vi "Test_HelloWorld_InvalidUtf8Encoding.vi"() -> (0 "Array of Error Description":T1)   [LabVIEW 2019]
uses:
  gRPC_ATS/TestUtility/utility.llb/array of error description.ctl
  gRPC_ATS/TestUtility/utility.llb/error description.ctl
  gRPC_ATS/TestUtility/utility.llb/error type.ctl
  examples/helloworld/helloworld_client/RPC Messages/helloworld_HelloRequest.ctl
  690210b7-9fc1-4805-899f-f09b8e1640af.vi
  86c0777a-bec3-4a03-9553-2f9525a5fa02.vi
  <vilib>/gRPC/LabVIEW gRPC Library/Server API/Translate Protobuf Error.vi
  <vilib>/AdvancedString/1D String Array to Delimited String.vi
  <vilib>/gRPC/LabVIEW gRPC Library/Server API/Server/Get Server DLL Path.vi
  examples/helloworld/helloworld_client/helloworld_client.lvlib
panel:
  out "Pass":bool
  in  "error in (no error)":errorcluster
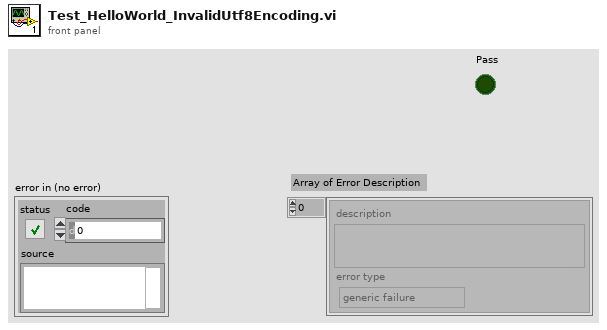
[diagram p1: front panel]
types:
  T1 = typedef "array of error description.ctl" = T2[]
  T2 = typedef "error description.ctl" = cluster{"description":string, "error type":T3}
  T3 = typedef "error type.ctl" = enum32{"generic failure", "boundary case", "precision", "expected error"}
  T4 = typedef "helloworld_client.lvlib/helloworld_HelloRequest.ctl" = cluster{"name":string}
  T5 = typedef "grpc-lvsupport-release.lvlib/grpcId.ctl" = u64
  T6 = typedef "grpc-lvsupport-release.lvlib/Any.ctl" = cluster{"Type Url":string, "Bytes":u8[]}
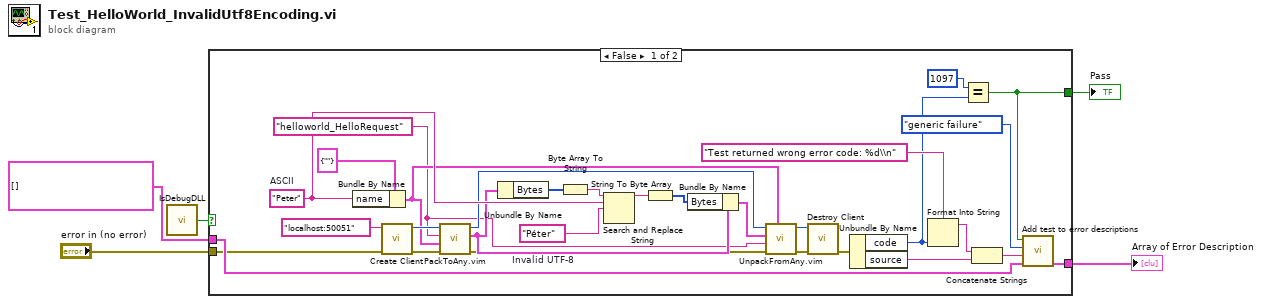
[diagram p0: block diagram]
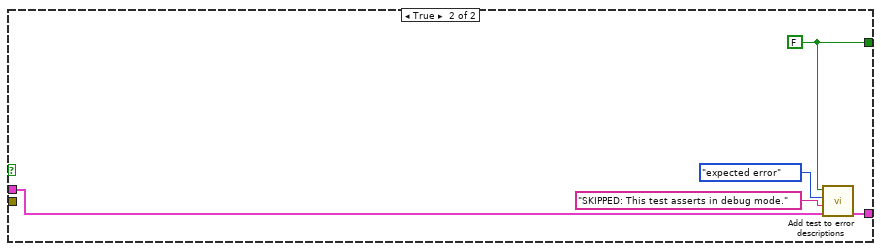
[diagram p2: hidden frame]
diagram:
  n1 = call "IsDebugDLL.vi"() -> ("is debug DLL?"=w1:bool)
  n2 = case shown="False" w1 {
    tunnel: T1 [] ("error descriptions in") -> [w35 w40]
    tunnel: [w34 w39] -> w4
    tunnel: "error in (no error)" -> [w13 _]
    tunnel: [w6 w36] -> w2
    frame False {
      w23 = "Péter"  # Invalid UTF-8
      w24 = "Peter"  # ASCII
      w16 = "helloworld_HelloRequest" ("Message Type")
      n3 = Bundle By Name(cluster=T4 {"name"=""} ("helloworld_HelloRequest"), "name"=w24) -> (w18:T4)
      n4 = call "Create Client.vi"("error in"=w13, "address"="localhost:50051") -> ("error out"=w30:errorcluster, "gRPC ID Out"=w29:T5)  [unwired: 8 in]
      n5 = call "PackToAny.vim"("error in"=w30, "Data To Pack"=w18, "Message Type"=w16, "gRPCid in"=w29) -> ("error out"=w14:errorcluster, "Any"=w21:T6, "gRPCid out"=w17:u64)  [unwired: 5 in]
      n6 = Unbundle By Name(w21) -> ("Bytes"=w26:u8[])
      n7 = Byte Array To String(unsigned byte array=w26) -> (string=w25:string)
      n8 = Search and Replace String(input string=w25, search string=w24, replace string=w23) -> (result string=w22:string)  [unwired: 5 in, 3 out]
      n9 = String To Byte Array(string=w22) -> (unsigned byte array=w20:u8[])
      n10 = Bundle By Name(cluster=w21, "Bytes"=w20) -> (w19:T6)
      n11 = call "UnpackFromAny.vim"("Data Type"=w18, "error in"=w14, "Message Type"=w16, "Any"=w19, "gRPCid in"=w17) -> ("error out"=w11:errorcluster, "gRPCid out"=w15:u64)  [unwired: 4 in, 1 out]
      n12 = call "Destroy Client.vi"("error in"=w11, "gRPC ID"=w15) -> ("error out"=w12:errorcluster)  [unwired: 9 in]
      n13 = Unbundle By Name(w12) -> ("code"=w8:i32, "source"=w32:string)
      n14 = Format Into String(format string="Test returned wrong error code: %d\\n" ("string"), w8) -> (resulting string=w7:string)  [unwired: 2 in, 1 out]
      n15 = Equal?(x=1097, y=w8) -> (x = y?=w6:bool)
      n16 = Concatenate Strings(w7, w32) -> (w33:string)
      n17 = call "Add test to error descriptions.vi"("error descriptions in"=w35, "error string"=w33, "error type"=error_type."generic failure", "pass"=w6) -> ("error description out"=w34:T1)  [unwired: 3 in]
    }
    frame True {
      w36 = FALSE ("pass")
      n18 = call "Add test to error descriptions.vi"("error descriptions in"=w40, "error string"="SKIPPED: This test asserts in debug mode.", "error type"=error_type."expected error", "pass"=w36) -> ("error description out"=w39:T1)  [unwired: 3 in]
    }
  }
  "Array of Error Description" <- w4
  "Pass" <- w2
